vi "Destroy User Events.vi"(11 "Configurator Actor:Configuration UI Actor in":refnum<class "Configuration UI Actor.lvclass">) -> (3 "Configurator Actor:Configuration UI Actor out":refnum<class "Configuration UI Actor.lvclass">)   [LabVIEW 2023, in "Configuration UI Actor.lvlib" / "Configuration UI Actor.lvclass"]
uses:
  Configuration UI Actor.lvclass
  Configuration UI Actor.lvclass/Configuration UI Actor.ctl
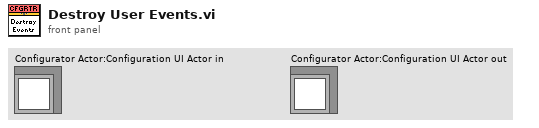
[diagram p1: front panel]
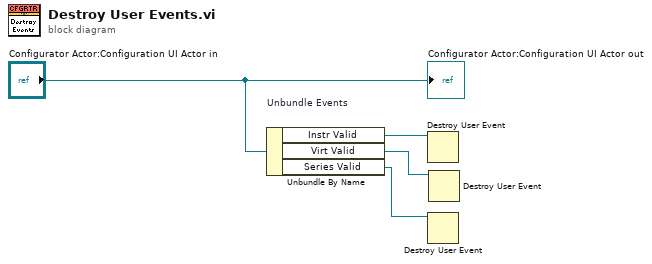
[diagram p0: block diagram]
diagram:
  n1 = Unbundle By Name "Unbundle Events"("Configurator Actor:Configuration UI Actor in") -> ("Instr Valid"=w3:refnum<user-event>, "Virt Valid"=w2:refnum<user-event>, "Series Valid"=w1:refnum<user-event>)
  n2 = Destroy User Event(user event=w3) -> ()  [unwired: 1 in, 1 out]
  n3 = Destroy User Event(user event=w1) -> ()  [unwired: 1 in, 1 out]
  n4 = Destroy User Event(user event=w2) -> ()  [unwired: 1 in, 1 out]
  "Configurator Actor:Configuration UI Actor out" <- "Configurator Actor:Configuration UI Actor in"
